vi "test count.vi"() -> ()   [LabVIEW 2019]
uses:
  cmd_count.ctl
panel:
  out "Array_data":dbl[][](array[numeric])
  in  "Array_Count":dbl[](array[numeric])
  in  "stop":bool
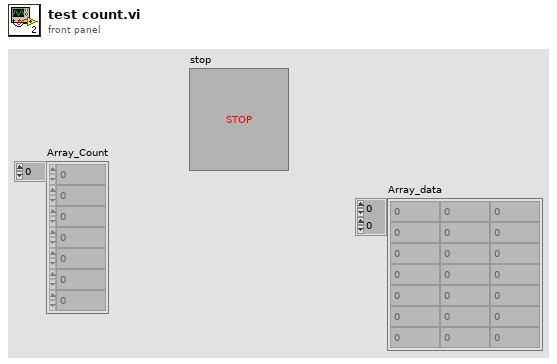
[diagram p1: front panel]
types:
  T1 = typedef "cmd_count.ctl" = enum16{"init", "count", "default"}
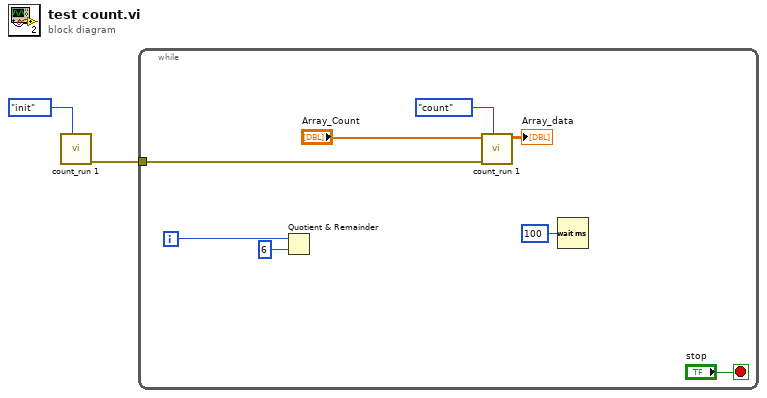
[diagram p0: block diagram]
diagram:
  n1 = call "count_run 1.vi"("cmd"=cmd_count."init") -> ("error out"=w1:errorcluster)  [unwired: 9 in, 1 out]
  n2 = while {
    tunnel: w1 -> [w8]
    i -> [w5]
    stop <- "stop" stop-if-true
    n3 = Quotient & Remainder(x=w5, y=6) -> ()  [unwired: 2 out]
    n4 = call "count_run 1.vi"("cmd"=cmd_count."count", "error in (no error)"=w8, "Array_Count"="Array_Count") -> ("Array_data"=→"Array_data":dbl[][])  [unwired: 7 in, 1 out]
    n5 = Wait (ms)(milliseconds to wait=u32 100) -> ()  [unwired: 1 out]
  }
